vi "MaskHandler.vi"(0 "UiDefinition 2":T1, 1 "Wafer Definition File":path, 2 "Save Wafer":bool, 5 "TestPointsLoaded in":bool, 7 "Load Mask":bool, 9 "Masks":string, 11 "dxfFile":string, 13 "WaferTestPoints":string) -> (4 "Path":path, 6 "TestPointsLoaded out":bool, 8 "body 2":string, 10 "body":string)   [LabVIEW 2020]
uses:
  UIReferences.ctl
  C:/Users/User/Desktop/Automation/CurrentVersion/LabviewDXFViewer/bin/Release/LabviewDXFViewer.exe
  LabviewDXFViewer/bin/Release/LabviewDXFViewer.exe
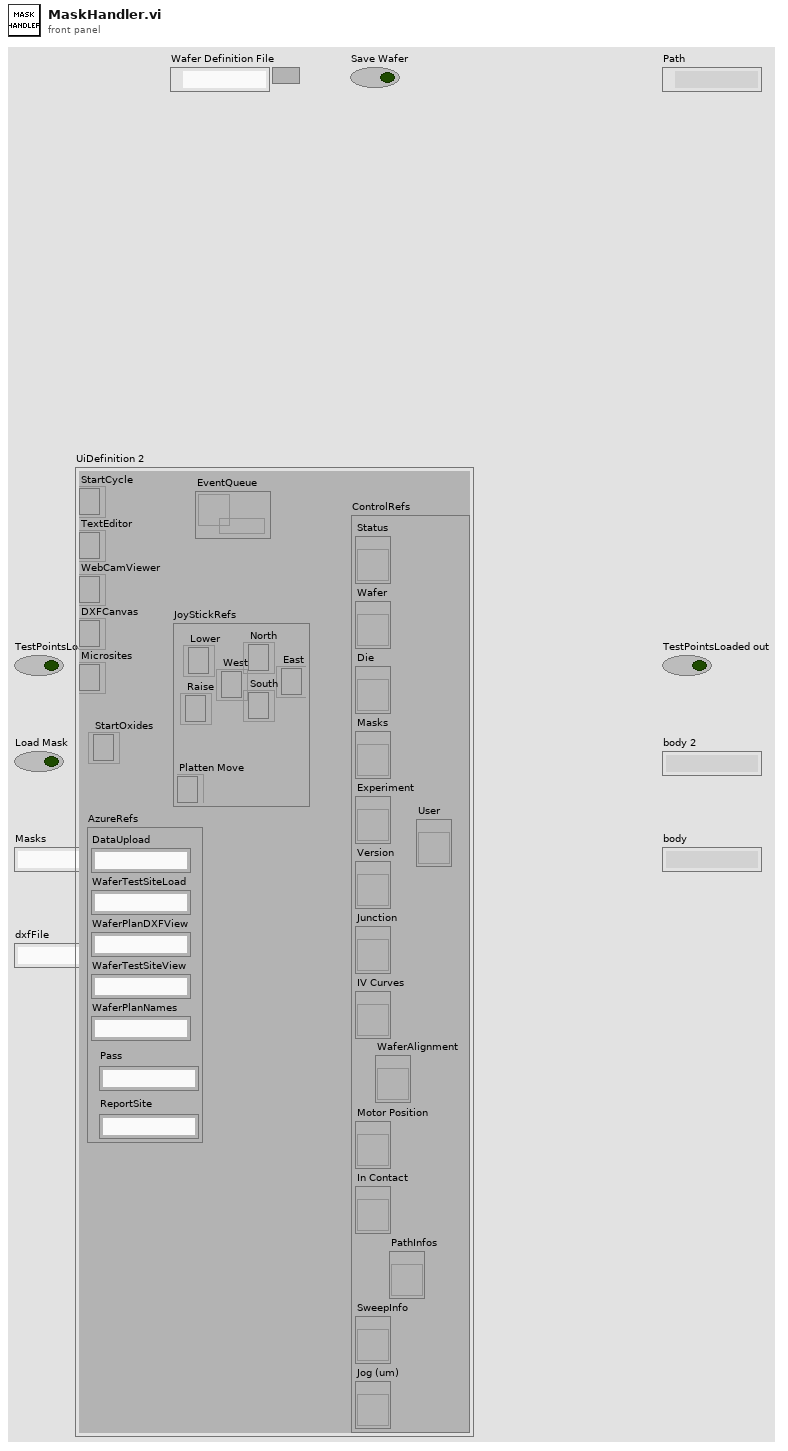
[diagram p1: front panel]
types:
  T1 = typedef "UIReferences.ctl" = cluster{"StartCycle":refnum<k24>, "TextEditor":refnum<k24>, "WebCamViewer":refnum<k24>, "DXFCanvas":refnum<k24>, "Microsites":refnum<k24>, "JoyStickRefs":cluster{"North":refnum<k24>, "Lower":refnum<k24>, "Raise":refnum<k24>, "Platten Move":refnum<k24>, "West":refnum<k24>, "East":refnum<k24>, "South":refnum<k24>}, "AzureRefs":cluster{"DataUpload":string, "WaferTestSiteLoad":string, "WaferPlanDXFView":string, "WaferTestSiteView":string, "WaferPlanNames":string, "Pass":string, "ReportSite":string}, "ControlRefs":cluster{"Status":refnum<vi>, "Wafer":refnum<vi>, "Die":refnum<vi>, "Masks":refnum<vi>, "Experiment":refnum<vi>, "Version":refnum<vi>, "Junction":refnum<vi>, "IV Curves":refnum<vi>, "Motor Position":refnum<vi>, "In Contact":refnum<vi>, "SweepInfo":refnum<vi>, "Jog (um)":refnum<vi>, "PathInfos":refnum<vi>, "User":refnum<vi>, "WaferAlignment":refnum<vi>}, "EventQueue":refnum<queue>, "StartOxides":refnum<k24>}
  T2 = cluster{"DataUpload":string, "WaferTestSiteLoad":string, "WaferPlanDXFView":string, "WaferTestSiteView":string, "WaferPlanNames":string, "Pass":string, "ReportSite":string}
  T3 = typedef "Control 2.ctl" = cluster{"Y":dbl[], "Current (A)":dbl[]}
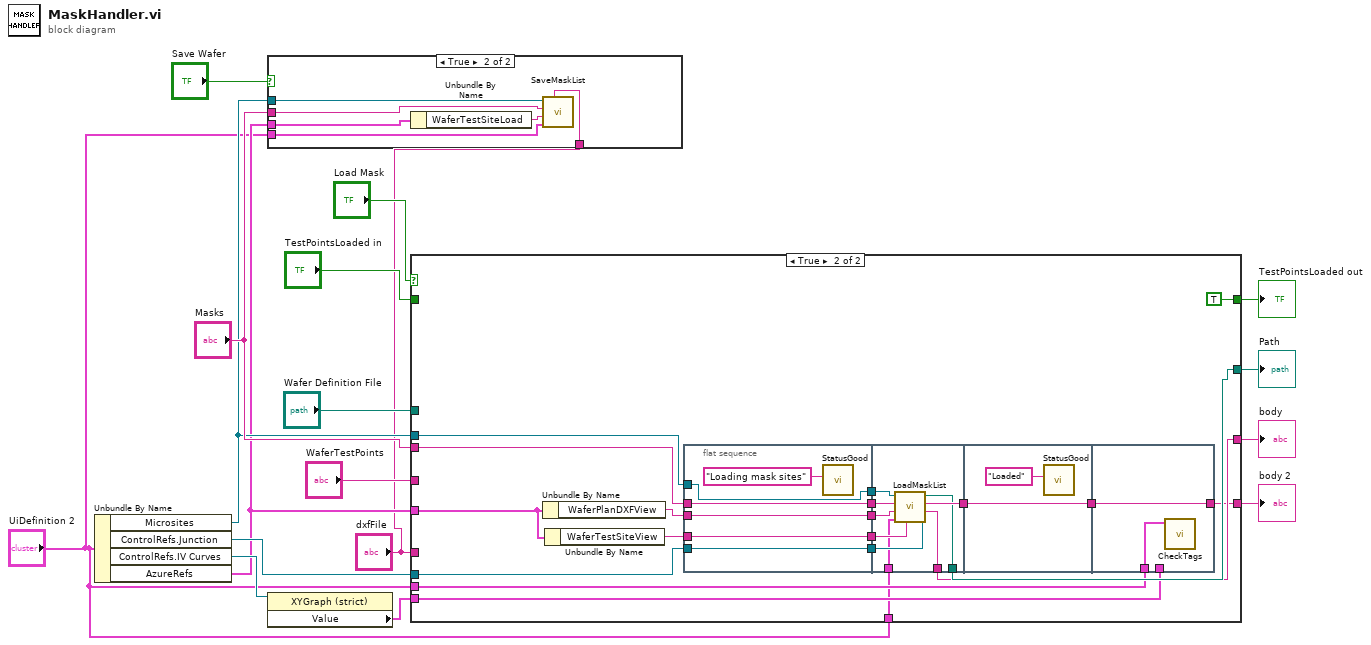
[diagram p0: block diagram]
diagram:
  n1 = Unbundle By Name("UiDefinition 2") -> ("Microsites"=w7:refnum<k24>, "ControlRefs.Junction"=w6:refnum<vi>, "ControlRefs.IV Curves"=w5:refnum<vi>, "AzureRefs"=w3:T2)
  n2 = case shown="True" "Save Wafer" {
    tunnel: "Masks" -> [_ w23]
    tunnel: w3 -> [_ w22]
    tunnel: w7 -> [_ w20]
    tunnel: "UiDefinition 2" -> [_ w19]
    tunnel: "dxfFile" -> [_ w18]
    frame False {
    }
    frame True {
      n3 = Unbundle By Name(w22) -> ("WaferTestSiteLoad"=w21:string)
      n4 = call "SaveMaskList.vi"("dxfFile"=w18, "UiDefinition 2"=w19, "url"=w21, "Masks"=w23, ".NET Refnum in"=w20) -> ()  [unwired: 7 in]
    }
  }
  n5 = property class="XYGraph (strict)"(reference=w5) -> ("Value"=w4:T3)  [unwired: 1 in, 2 out]
  n6 = case shown="True" "Load Mask" {
    tunnel: "Masks" -> [_ w47]
    tunnel: w3 -> [_ w46]
    tunnel: w6 -> [_ w45]
    tunnel: [w27 TRUE] -> w11
    tunnel: "TestPointsLoaded in" -> [w27 _]
    tunnel: [w26 w34] -> w13
    tunnel: [w25 w33] -> w14
    tunnel: "Wafer Definition File" -> [w26 _]
    tunnel: "WaferTestPoints" -> [w25 _]
    tunnel: w4 -> [_ w32]
    tunnel: [w24 w31] -> w17
    tunnel: "dxfFile" -> [w24 _]
    tunnel: w7 -> [_ w30]
    tunnel: "UiDefinition 2" -> [_ w29]
    tunnel: "UiDefinition 2" -> [_ w28]
    frame False {
    }
    frame True {
      n7 = Unbundle By Name(w46) -> ("WaferPlanDXFView"=w44:string)
      n8 = Unbundle By Name(w46) -> ("WaferTestSiteView"=w43:string)
      n9 = flat-sequence {
        tunnel: w43 -> [w49]
        tunnel: w44 -> [w50]
        tunnel: w30 -> [w51]
        tunnel: w45 -> [w52]
        tunnel: w47 -> [w53]
        tunnel: [w53] -> w42
        tunnel: [w52] -> w41
        tunnel: [w51] -> w40
        tunnel: [w50] -> w39
        tunnel: [w49] -> w38
        tunnel: w42 -> [w61]
        tunnel: w41 -> [w60]
        tunnel: w40 -> [w59]
        tunnel: w39 -> [w58]
        tunnel: w38 -> [w57]
        tunnel: [w56] -> w34
        tunnel: [w55] -> w33
        tunnel: [w62] -> w37
        tunnel: w28 -> [w54]
        tunnel: w37 -> [w64]
        tunnel: [w64] -> w36
        tunnel: [w66] -> w31
        tunnel: w36 -> [w66]
        tunnel: w32 -> [_]
        tunnel: w29 -> [w65]
        frame #0 {
          n10 = call "StatusGood.vi"("Text.Text"="Loading mask sites") -> ()  [unwired: 11 in]
        }
        frame #1 {
          n11 = call "LoadMaskList.vi"("JunctionList"=w60, "url 2"=w57, "UiDefinition 2"=w54, "url"=w58, "Masks"=w61, "Microsites ref"=w59) -> ("body"=w55:string, "body 2"=w62:string, "Path"=w56:path)  [unwired: 3 in]
        }
        frame #2 {
          n12 = call "StatusGood.vi"("Text.Text"="Loaded") -> ()  [unwired: 11 in]
        }
        frame #3 {
          n13 = call "CheckTags.vi"("UiDefinition 2"=w65) -> ()  [unwired: 10 in, 1 out]
        }
      }
    }
  }
  "body 2" <- w17
  "body" <- w14
  "Path" <- w13
  "TestPointsLoaded out" <- w11
